vi "Simulador_PID.vi"() -> ()   [LabVIEW 2013]
uses:
  <vilib>/Simulation/Scripting/Companion Diagram/SimConfigNode/SimParams.ctl
  <vilib>/Simulation/Scripting/Companion Diagram/SimConfigNode/_simSolvers.ctl
  <vilib>/Simulation/Implementation/Shared/SIMSCR Execution Mode.ctl
  <vilib>/Simulation/Param Hierarchy/Typedefs/SIMPH Param Control Actions.ctl
  <vilib>/Simulation/Implementation/Shared/SIM limit type.ctl
  <vilib>/Simulation/Scripting/Editor Utilities/SIM subVI tag data.ctl
  <vilib>/Simulation/Scripting/Editor Utilities/SIM subVI execution type.ctl
  <vilib>/Simulation/Implementation/Shared/NILVSim_ParamChanged.vi
  <vilib>/Simulation/Implementation/Shared/NILVSIM_BeginStep.vi
  <vilib>/Simulation/ContinuousLinear/Implementation/NILVSim Transfer Function.llb/SIM Transfer Function Distributor (SISO CD).vi
  <vilib>/Simulation/ContinuousLinear/Implementation/NILVSim Integrator new.llb/SIM Integrator distributor (scalar).vi
  <vilib>/Simulation/Implementation/Shared/SIM Fire Discrete SubVI.vi
  <vilib>/Simulation/SignalArithmetic/Implementation/NILVSim Gain.llb/SIM Gain (scalar).vi
  <vilib>/Simulation/Nonlinear/Implementation/NILVSim Saturation.llb/SIM Saturation (scalar).vi
  <vilib>/Simulation/ContinuousLinear/Implementation/NILVSim Transfer Function.llb/SIM Transfer Function Collector (SISO).vi
  <vilib>/Simulation/SignalDisplay/Implementation/NILVSim Time Waveform.llb/SIM Time Waveform (scalar).vi
  <vilib>/Simulation/ContinuousLinear/Implementation/NILVSim Integrator new.llb/SIM Integrator collector (scalar).vi
  <vilib>/Simulation/Implementation/Shared/NILVSim_Manager.vi
  <vilib>/Simulation/Implementation/Shared/NILVSim_FinalizeModel.vi
  <vilib>/Simulation/Implementation/Shared/SIM Fire Discrete SubVI (Core).vi
  <vilib>/Simulation/Implementation/Shared/SIM Unbundle Sim Info.vi
  <vilib>/Utility/error.llb/Clear Errors.vi
  <vilib>/Simulation/Implementation/Shared/NILVSim_GetModelError.vi
  <vilib>/Simulation/Implementation/Shared/SIM Bundle Sim Info.vi
  <vilib>/Simulation/Implementation/Shared/SIMSH Read Queue.vi
  <vilib>/Simulation/Implementation/Shared/NILVSim_Initialize.vi
  <vilib>/addons/Control Design/_Model Construction/Model Creation.llb/CD Construct Transfer Function Model.vi
  <vilib>/addons/Control Design/_Model Construction/Model Creation.llb/Model Creation SubVI/cd_Create Transfer Function Model.vi
  <vilib>/Simulation/Utility/Implementation/NILVSim Get Time and IsAcceptedStep.vi
  <vilib>/Simulation/Scripting/Companion Diagram/SimConfigNode/SimDog.xnode
  <vilib>/Simulation/Implementation/XNodeFramework/SimXNode/SimX.xnode
  <vilib>/Simulation/ContinuousLinear/Implementation/NILVSim Integrator new.llb/SIM Integrator (scalar).vi
  <vilib>/addons/Control Design/_Model Construction/Model Typedefs.llb/CD Transfer Function Model (SISO).ctl
  <vilib>/addons/Control Design/_Model Construction/NI_LinSys_Model Typedefs.lvlib
  <vilib>/addons/Control Design/_Model Construction/Model Typedefs.llb/CD General Elements.ctl
  <vilib>/addons/Control Design/_Model Construction/Model Typedefs.llb/CD Transfer Function Model (MIMO).ctl
  <vilib>/addons/Control Design/_Model Construction/NI_LinSys_Model Creation.lvlib
  <vilib>/Simulation/ContinuousLinear/Implementation/NILVSim Transfer Function.llb/SIM Transfer Function (SISO CD).vi
  <vilib>/Simulation/Implementation/Shared/NI_SIM_Implementation.lvlib
panel:
  in  "K":dbl=0.6
  in  "Tau":dbl=37.15
  in  "stop":bool
  in  "Kp":dbl=2.271
  in  "Ki":dbl=0.0627
  in  "SV":dbl=60.0
  out "Resposta degrau":waveform(dbl)(graph)
  out "Sinal de controle[%]":waveform(dbl)(graph)
  in  "Simulate":bool
  in  "Tamb":dbl=26.0
  in  "Theta":dbl=26.6
  # "Inserir dados da planta"
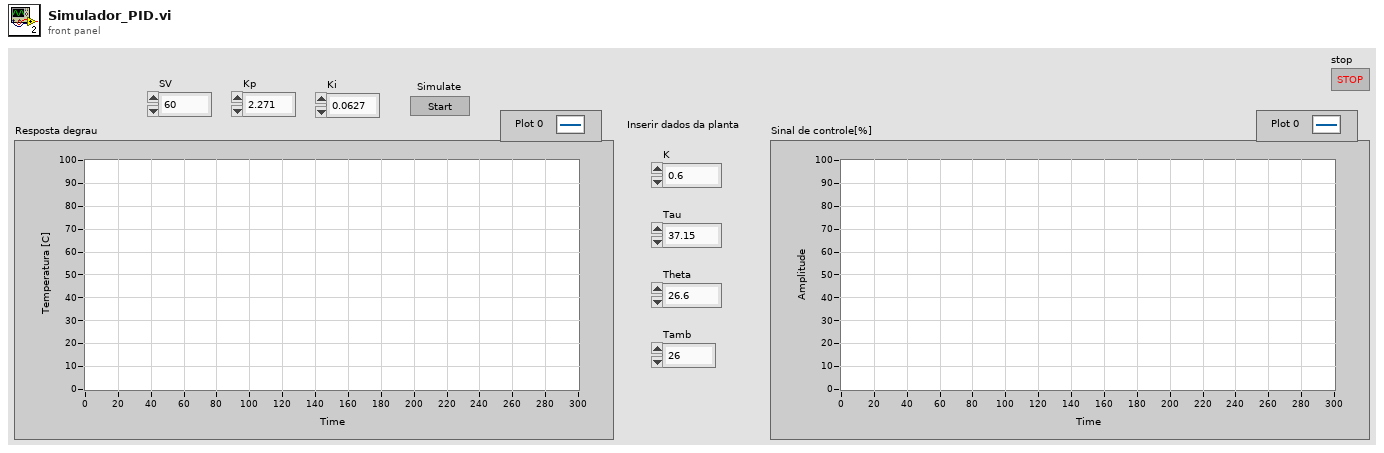
[diagram p1: front panel]
types:
  T1 = typedef "SIMSCR Execution Mode.ctl" = enum16{"Simulate to Completion", "Single Time-Step Simulation (Fixed Step Only)"}
  T2 = typedef "SIMPH Param Control Actions.ctl" = enum16{"get params", "set params"}
  T3 = typedef "SIM subVI tag data.ctl" = cluster{"period":dbl, "skew":dbl, "Simulation execution type":T4}
  T4 = typedef "SIM subVI execution type.ctl" = enum16{"Function call", "Discrete", "Continuous", "Initialization only", "Final step only"}
  T5 = typedef "SIM limit type.ctl" = enum16{"upper", "lower", "both", "none"}
  T6 = typedef "SimParams.ctl" = cluster{"Initial Time (s)":dbl, "Final Time (s)":dbl, "Step Size (s)":dbl, "ODE Solver":T7, "Minimum Step Size (s)":dbl, "Maximum Step Size (s)":dbl, "Relative Tolerance":dbl, "Absolute Tolerance":dbl, "Software Timing":bool, "Initial Step Size (s)":dbl, "Automatic Fixed Step Size?":bool, "Automatic Discrete Step Size?":bool, "Discrete Step Size (s)":dbl, "Calculate using Time Step":bool, "Solver Wired?":bool, "Prev.Frm.Expected End":u64, "Prev.Frm.Actual End":u64, "Prev.Frm.Finished Late?":bool, "Prev.Iter.Expected End":u64, "Prev.Iter.Actual End":u64, "Prev.Iter.Finished Late?":bool, "Expected Iteration Start":u64, "Actual Iteration Start":u64, "Expected Frame Start":u64, "Actual Frame Start":u64, "Source Name":string, "Name":string, "Period":i64, "Deadline":i64, "Offset":i64, "Start":i64, "Priority":i32, "Timeout":i32, "Processor":i32, "Mode":enum32{"No Change", "Process missed periods, maintain original phase", "Discard missed periods, maintain original phase", "Process missed periods, ignore original phase", "Discard missed periods, ignore original phase"}, "Wakeup reason":enum32{"Normal", "Aborted", "Asynchronous wakeup", "Timing source error", "Timed loop error", "Timeout"}, "Error":errorcluster, "Source Type":string, "Secondary Source Type":string, "Global End Time":u64, "Global Start Time":u64, "Full Solver Reset":bool, "Execution Mode":T1, "Nan/Inf Check":bool, "Custom Solver Library":string, "Solver Is Variable":bool, "custom solver name":string, "Signal Collection Decimation":u32}
  T7 = typedef "_simSolvers.ctl" = enum16{"Runge-Kutta 1 (Euler)", "Runge-Kutta 2", "Runge-Kutta 3", "Runge-Kutta 4", "Runge-Kutta 23 (variable)", "Runge-Kutta 45 (variable)", "BDF (variable)", "Adams-Moulton (variable)", "Rosenbrock (variable)", "Discrete States Only", "SDIRK 4 (variable)", "Radau 5 (variable)", "Radau 9 (variable)", "Radau 13 (variable)", "Radau [Variable Order] (variable)", "Gear's Method (variable)", "Linearizer", "State Query", "Trim Eval", "Custom Solver"}
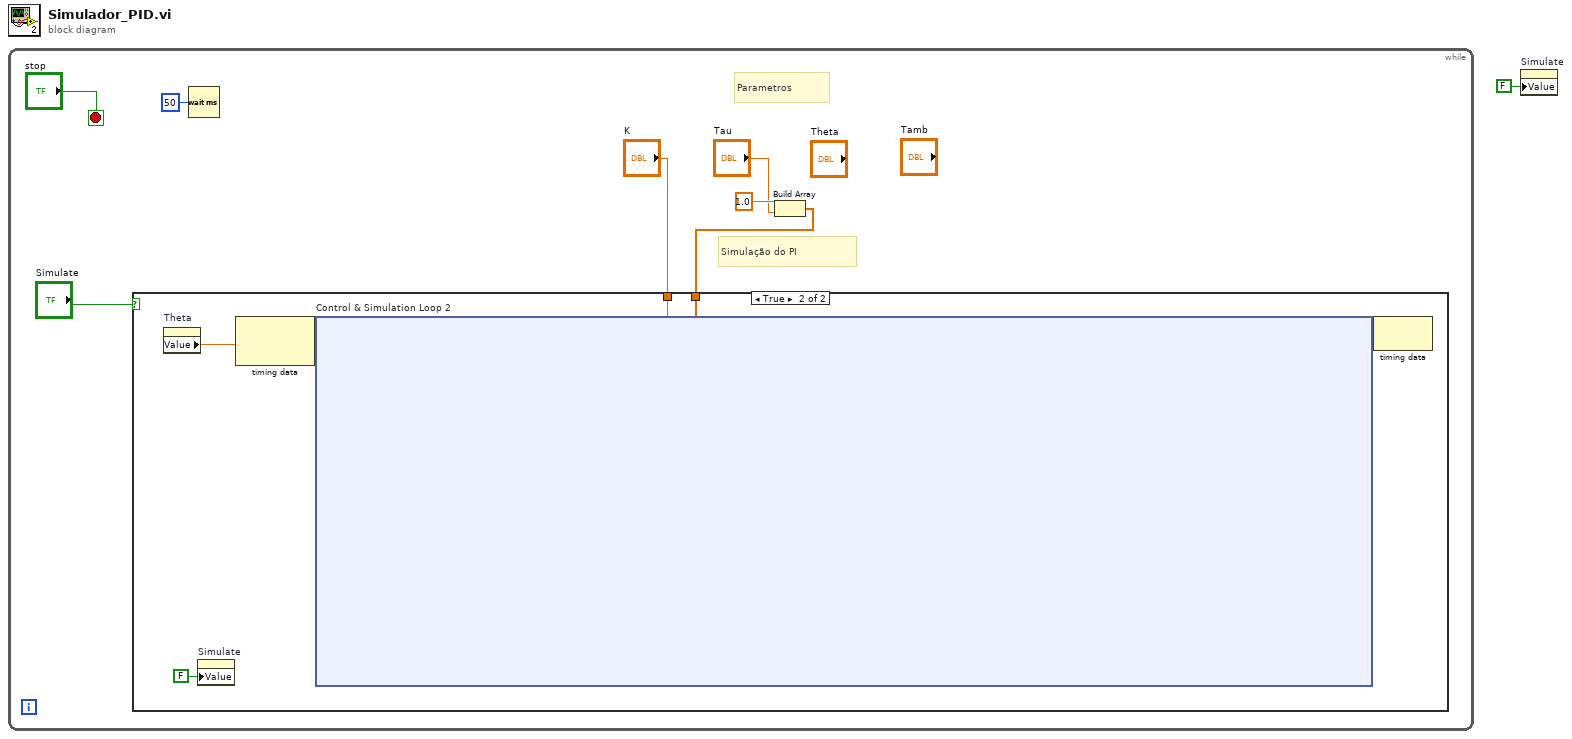
[diagram p0: block diagram]
diagram:
  n1 = while {
    stop <- "stop" stop-if-true
    # "Simulação do PI"
    # "Parametros"
    n2 = Wait (ms)(milliseconds to wait=u32 50) -> ()  [unwired: 1 out]
    n3 = Build Array(1.0 ("element"), "Tau") -> (w2:dbl[])
    n4 = case shown="True" "Simulate" {
      tunnel: "K" -> [_ w10]
      tunnel: w2 -> [_ w9]
      frame False {
      }
      frame True {
        n5 = property on="Theta" class="DigNum (strict)"() -> ("Value"=w11:dbl)  [unwired: 2 in, 2 out]
        n6 = property on="Simulate" class="Bool (strict)"("Value"=FALSE ("Simulate")) -> ()  [unwired: 2 in, 2 out]
        n7 = node-c288(w11) -> (w14:variant)  [unwired: 1 in]
        n8 = node-c254 "Control & Simulation Loop 2"(w14, w10, w9) -> (w13:variant)
        n9 = node-c288(w13) -> ()  [unwired: 1 out]
      }
    }
  }
  n10 = property on="Simulate" class="Bool (strict)"("Value"=FALSE ("Simulate")) -> ()  [unwired: 2 in, 2 out]
